vi "keeperStuck.vi"(8 "error in (no error)":errorcluster, 9 "Game":refnum<class "Game.lvclass">, 10 "Robot in":refnum<class "Robot.lvclass">, 11 "DefendGoalTactic in":refnum<class "DefendGoalTactic.lvclass">) -> (0 "error out":errorcluster, 2 "kepperStuck":bool, 3 "DefendGoalTactic out":refnum<class "DefendGoalTactic.lvclass">)   [LabVIEW 2024, in "DefendGoalTactic.lvclass"]
uses:
  DefendGoalTactic.lvclass
  Robot_class/Robot.lvclass
  Game_class/Game.lvclass
  Game_class/Game.lvclass/Game.ctl
  Object_class/Object.lvclass/Object.ctl
  Game_class/Read NewParameters.vi
  Game_class/Read FieldRef.vi
  Game_class/Read BallRef.vi
  Object_class/Read y.vi
  Object_class/Read x.vi
  Ball_class/Ball.lvclass
  C:/Users/ROBOIME2/Documents/SSL ROBOIME/SSL_AI/Object_class/Object.lvclass
  Field_class/Field.lvclass
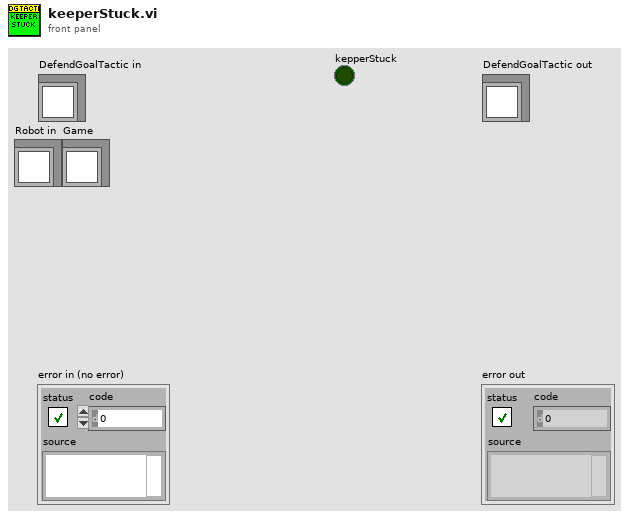
[diagram p1: front panel]
types:
  T1 = typedef "NewParameters.ctl" = cluster{"PenaltyDistance":dbl, "DistanceAttackerToBackBall":dbl, "Division":enum16{"Div B", "Div A"}, "DistanceToAvoidyEnemyRobot":dbl, "BallPlacementDistance":dbl, "DisatanceBehindBallToStealBall":dbl, "MaxDistanceToPositionKickoff":dbl, "BlockEnemyTarget":bool, "MaxStopVAng":dbl, "DistanceMarkerToEnemy":dbl, "IgnoreDribblerContact":bool, "DistanceToBeginEnemyPosession":dbl, "GoToBallWhenEnemyNotMoving":bool, "EnemyDistanceToReduceVelocity":dbl, "TurnOnEnemyDistanceToReduceVelocity":bool, "EnemyDistanceToShootOutBall":dbl, "DefenseKickBall":bool, "MoreKickToGoal? (0-0.3)":dbl, "ChipKickInEnemyField":bool, "ShootOutRobotId":dbl, "FieldLenghtDenominatorInShootOut":dbl, "AdjustPositionInBallPlacement":bool, "PowerGodPass":dbl, "VelocityAbortEnemyPos":dbl, "MaxDistToBeginPass":dbl, "MinDistToBeginPass":dbl, "VelocityInDirects":dbl, "BadDribblerIDs":i32[], "NewKickToDistanceAroundBall":dbl, "PowerAvoidColisionMarker":dbl, "DistanceToAvoidColisionMarker":dbl, "AvoidBallKick":dbl, "DistanceTryKick":dbl, "SuicideKickDIstance":dbl, "AdjustFirstKickDistance":dbl, "AvoidAimLessKick":dbl, "DistanceToAvoidyEnemyShootRobot ":dbl, "NumberOfMarkers":dbl, "PotField":bool, "PIDLateral":bool, "MinDistanceFirstKickX":dbl, "MinDistanceFirstKickY":dbl, "FractionOfDistToTouchGround\nAfterChipKick":dbl, "FractionOfKickxWhen\nComposedWithKickz":dbl, "Style":T2, "MoveInTurnState":bool, "DistFromEnemyToConsider\nMoveInTurnState":dbl, "CascadePID":bool, "TurnAroundParameters":cluster{"Radius":dbl, "Multiplier":dbl, "ChordAngle":dbl}, "SafeDriveVel":dbl, "DistanceToGoToBackBall":dbl, "minDistanceToNotFinish\nEnemyPossession":dbl, "OneTouchShot":cluster{"angleFactor":dbl, "maxAngle":dbl, "Attack":bool, "Defense":bool}, "OpenAngleToGoal":cluster{"minAngle":dbl, "maxAngle":dbl, "minEvaluation":dbl}, "ShotInterception":cluster{"shotSpeed":dbl, "minEnemySpeed":dbl, "maxEnemySpeed":dbl, "minEvaluation":dbl}, "AllyTeamArray":T3[], "maxDefendersNumber":i32, "Zone":cluster{"GuardPositionArray":dbl[][], "ZoneMidField":dbl[], "CenterForwardWidth":dbl}, "MinEvaluationToShoot":dbl, "PassInterception":cluster{"maxPassSpeed":dbl, "minPassSpeed":dbl, "minEnemySpeed":dbl, "chipPassDistance":dbl, "chipPassEvaluation":dbl, "minEvaluation":dbl, "maxEnemySpeed":dbl}, "PassDistance":cluster{"maxDistance":dbl, "minDistance":dbl}, "receiverSpeed":dbl, "maxBallSpeed":dbl, "slackTime":dbl, "Turning radius":dbl, "Turning v_ang":dbl, "AlignError":cluster{"Distance":dbl, "Orientation":dbl, "V_norm(m/s)":dbl, "V_ang (rad/s)":dbl}, "RobotRadius":dbl, "KickerDistance":dbl, "keeper angle  to cover goalpost":dbl, "a_slide":dbl, "a_roll":dbl, "k_switch":dbl}
  T2 = typedef "Style.ctl" = enum16{"Insanity", "Offensive", "Defensive"}
  T3 = typedef "AllyTeam.ctl" = enum16{"Keeper", "Defender", "Attacker"}
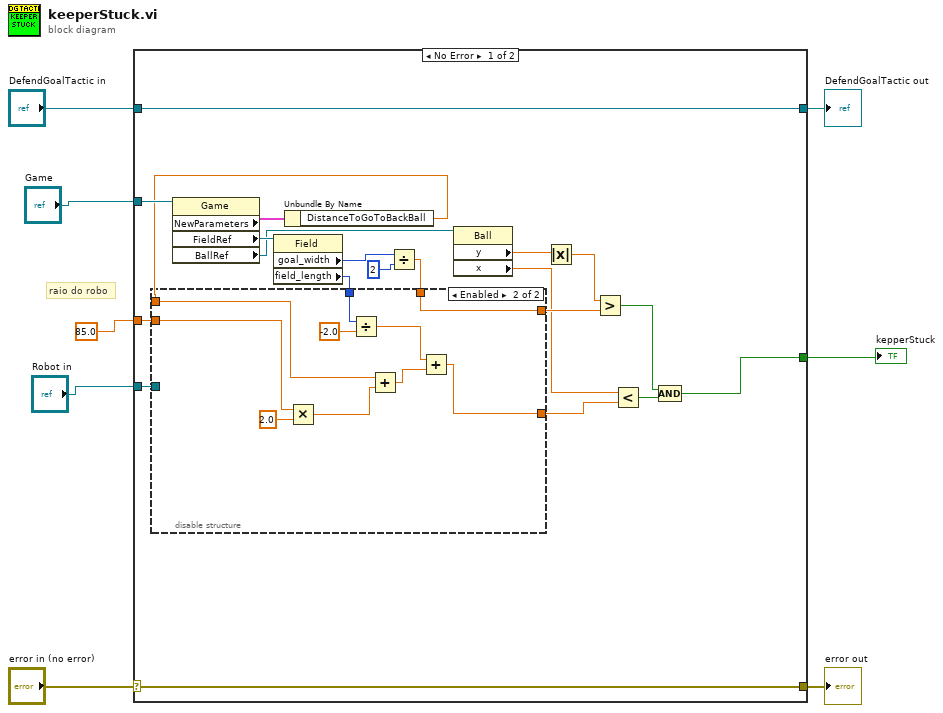
[diagram p0: block diagram]
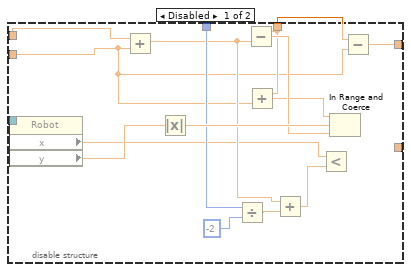
[diagram p2: hidden frame]
diagram:
  # "raio do robo"
  n1 = case shown="No Error" "error in (no error)" {
    selector: "error in (no error)" -> [w28 w56]
    tunnel: [w28 w56] -> w7
    tunnel: [w29 w55] -> w5
    tunnel: "DefendGoalTactic in" -> [w29 w55]
    tunnel: "Robot in" -> [w26 _]
    tunnel: "Game" -> [w27 _]
    tunnel: [w21 _] -> w2
    tunnel: 85.0 -> [w12 _]
    frame No Error {
      n2 = property class="Game"(reference=w27) -> ("NewParameters"=w23:T1, "FieldRef"=w25:refnum<class "Field.lvclass">, "BallRef"=w20:refnum<class "Ball.lvclass">)  [unwired: 1 in, 2 out]
      n3 = property class="Field"(reference=w25) -> ("goal_width"=w15:i32, "field_length"=w24:i32)  [unwired: 1 in, 2 out]
      n4 = Unbundle By Name(w23) -> ("DistanceToGoToBackBall"=w22:dbl)
      n5 = Divide(x=w15, y=2) -> (x/y=w13:dbl)
      n6 = disable-structure shown="Enabled" {
        disable-tunnel: w26 -> [w44 _]
        disable-tunnel: w24 -> [w39 w48]
        disable-tunnel: w22 -> [w33 w50]
        disable-tunnel: [w32 w54] -> w17
        disable-tunnel: w13 -> [w31 w54]
        disable-tunnel: w12 -> [w30 w52]
        disable-tunnel: [_ w45] -> w9
        frame Disabled {
          n7 = property class="Robot"(reference=w44) -> ("x"=w34:dbl, "y"=w40:dbl)  [unwired: 1 in, 2 out]
          n8 = Add(x=w33, y=w30) -> (x+y=w36:dbl)
          n9 = Absolute Value(x=w40) -> (abs(x)=w43:dbl)
          n10 = Divide(x=w39, y=-2) -> (x/y=w37:dbl)
          n11 = Subtract(x=w31, y=w36) -> (x-y=w42:dbl)
          n12 = Add(x=w31, y=w30) -> (x+y=w41:dbl)
          n13 = Add(x=w36, y=w37) -> (x+y=w35:dbl)
          n14 = Less?(x=w34, y=w35) -> ()  [unwired: 1 out]
          n15 = In Range and Coerce(upper limit=w41, x=w43, lower limit=w42) -> ()  [unwired: 2 out]
          n16 = Subtract(x=w31, y=w30) -> (x-y=w32:dbl)
        }
        frame Enabled {
          n17 = Multiply(x=w52, y=2.0) -> (x*y=w51:dbl)
          n18 = Divide(x=w48, y=-2.0) -> (x/y=w46:dbl)
          n19 = Add(x=w50, y=w51) -> (x+y=w47:dbl)
          n20 = Add(x=w46, y=w47) -> (x+y=w45:dbl)
        }
      }
      n21 = property class="Ball"(reference=w20) -> ("y"=w19:dbl, "x"=w10:dbl)  [unwired: 1 in, 2 out]
      n22 = Absolute Value(x=w19) -> (abs(x)=w18:dbl)
      n23 = Greater?(x=w18, y=w17) -> (0:w16:bool)
      n24 = Less?(x=w10, y=w9) -> (x < y?=w11:bool)
      n25 = Compound Arithmetic op=AND(w16, w11) -> (w21:bool)
    }
    frame Error {
    }
  }
  "error out" <- w7
  "DefendGoalTactic out" <- w5
  "kepperStuck" <- w2
